vi "Pre-Install Custom Action.vi"(10 "Variant":variant) -> (0 "error out":errorcluster)   [LabVIEW 2015]
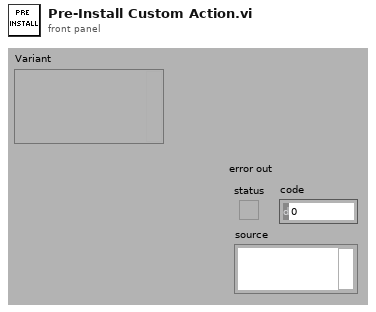
[diagram p1: front panel]
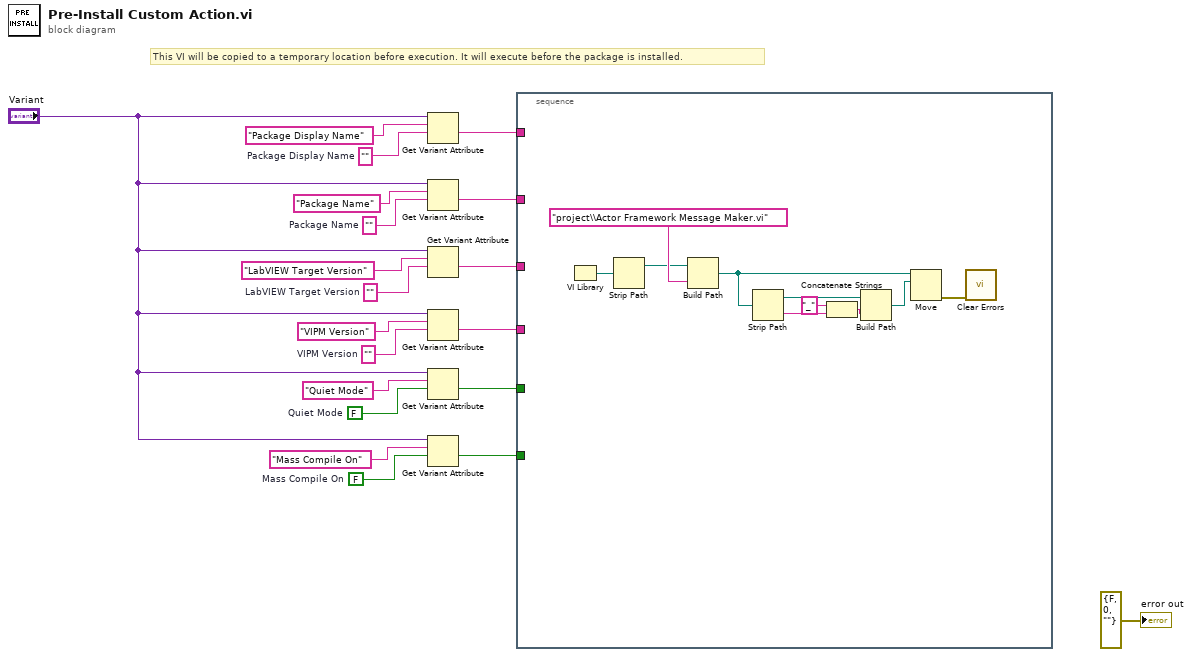
[diagram p0: block diagram]
diagram:
  w1 = FALSE  # Mass Compile On
  w3 = ""  # Package Display Name
  w10 = FALSE  # Quiet Mode
  w13 = ""  # VIPM Version
  w15 = ""  # LabVIEW Target Version
  w17 = ""  # Package Name
  # "This VI will be copied to a temporary location before execution. It will execute before the package is installed."
  n1 = Get Variant Attribute(Variant="Variant", name="Package Display Name", default value (empty Variant)=w3) -> (value=w9:string)  [unwired: 1 in, 3 out]
  n2 = Get Variant Attribute(Variant="Variant", name="Package Name", default value (empty Variant)=w17) -> (value=w8:string)  [unwired: 1 in, 3 out]
  n3 = Get Variant Attribute(Variant="Variant", name="LabVIEW Target Version", default value (empty Variant)=w15) -> (value=w7:string)  [unwired: 1 in, 3 out]
  n4 = Get Variant Attribute(Variant="Variant", name="VIPM Version", default value (empty Variant)=w13) -> (value=w6:string)  [unwired: 1 in, 3 out]
  n5 = Get Variant Attribute(Variant="Variant", name="Quiet Mode", default value (empty Variant)=w10) -> (value=w5:bool)  [unwired: 1 in, 3 out]
  n6 = Get Variant Attribute(Variant="Variant", name="Mass Compile On", default value (empty Variant)=w1) -> (value=w4:bool)  [unwired: 1 in, 3 out]
  n7 = stacked-sequence {
    tunnel: w9 -> [_]
    tunnel: w8 -> [_]
    tunnel: w7 -> [_]
    tunnel: w6 -> [_]
    tunnel: w5 -> [_]
    tunnel: w4 -> [_]
    frame #0 {
      n8 = VI Library() -> (path=w30:path)
      n9 = Strip Path(path=w30) -> (stripped path=w28:path)  [unwired: 1 out]
      n10 = Build Path(base path=w28, name or relative path="project\\Actor Framework Message Maker.vi") -> (appended path=w26:path)
      n11 = Strip Path(path=w26) -> (stripped path=w25:path, name=w24:string)
      n12 = Concatenate Strings("_" ("string"), w24) -> (w23:string)
      n13 = Build Path(base path=w25, name or relative path=w23) -> (appended path=w21:path)
      n14 = Move(source path=w26, 10:w21) -> (error out=w27:errorcluster)  [unwired: 3 in, 2 out]
      n15 = call <vilib>:"Clear Errors.vi"("error in (no error)"=w27) -> ()  [unwired: 5 in, 2 out]
    }
  }
  "error out" <- errorcluster {"status"=FALSE, "code"=0, "source"=""} ("error out")
